vi "Dereferncing 1D Array Pointer DBL.vi"(8 "error in (no error)":errorcluster, 10 "1D Double Array Pointer":u64, 11 "numberOfSamples":u32) -> (0 "error out":errorcluster, 3 "Array Data":dbl[](array[numeric]))   [LabVIEW 2022 SP3, in "MU_3SL_interface.lvlib"]
uses:
  MU_3SL_interface.lvlib
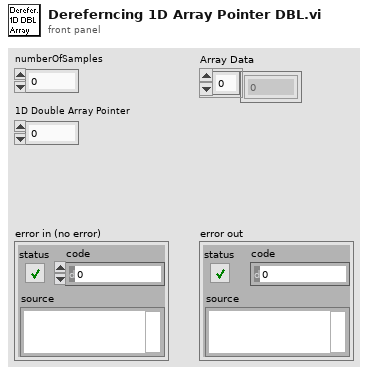
[diagram p1: front panel]
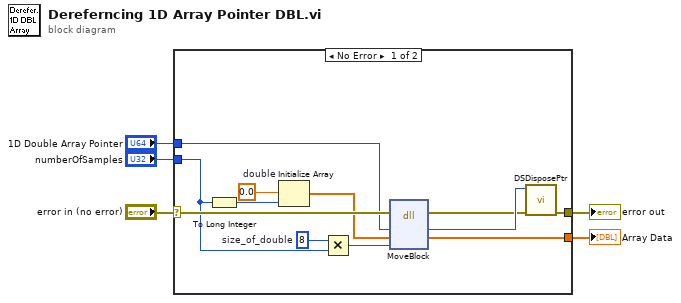
[diagram p0: block diagram]
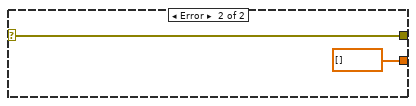
[diagram p2: hidden frame]
diagram:
  n1 = case shown="No Error" "error in (no error)" {
    selector: "error in (no error)" -> [w16 w19]
    tunnel: "numberOfSamples" -> [w7 _]
    tunnel: "1D Double Array Pointer" -> [w15 _]
    tunnel: [w17 w19] -> w4
    tunnel: [w10 dbl[] [] ("dest")] -> w3
    frame No Error {
      w8 = 0.0  # double
      w14 = u32 8  # size_of_double
      n2 = To Long Integer(number=w7) -> (32bit integer=w6:i32)
      n3 = Initialize Array(w8, w6) -> (w9:dbl[])
      n4 = Multiply(x=w14, y=w7) -> (x*y=w13:u32)
      n5 = dll-call lib="LabVIEW" fn="MoveBlock"(error in=w16, "source"=w15, "dest"=w9, "size"=w13) -> (error out=w11:errorcluster, "source"=w12:i64, "dest"=w10:dbl[])  [unwired: 4 in, 1 out]
      n6 = call <vilib>:"DSDisposePtr.vi"("error in (no error)"=w11, "Pointer"=w12) -> ("error out"=w17:errorcluster)  [unwired: 9 in]
    }
    frame Error {
    }
  }
  "error out" <- w4
  "Array Data" <- w3
